vi "Read Boolean Configuration.vi"(8 "error in (no error)":errorcluster, 9 "Default If Not Found":bool, 10 "Name":string, 11 "database-configuration in":refnum<class "configuration-database.lvclass">) -> (0 "error out":errorcluster, 1 "Not Found?":bool, 2 "Value":bool, 3 "database-configuration out":refnum<class "configuration-database.lvclass">)   [LabVIEW 2020, in "configuration-database.lvlib" / "configuration-database.lvclass"]
uses:
  configuration-database.lvclass
  configuration-database.lvclass/configuration-database.ctl
  bde3cf0d-0dad-4714-9e3b-43a1a7f5128d.vi
  bde3cf0d-0dad-4714-9e3b-43a1a7f5128d.vi/28ee1364-3f60-465d-b3c8-c72d5691017c.vi
  <vilib>/Utility/error.llb/Error Cluster From Error Code.vi
  IConfigDBQueries/IConfigurationDatabaseQueries.lvclass
  externals/database-interface/IDatabase/IDatabase/IDatabase.lvclass
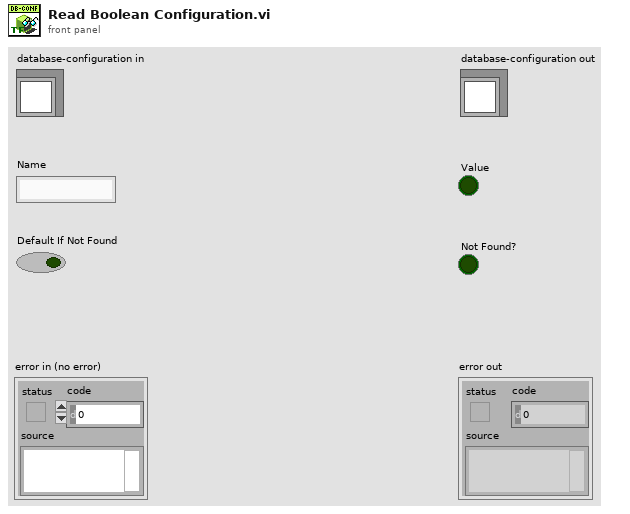
[diagram p1: front panel]
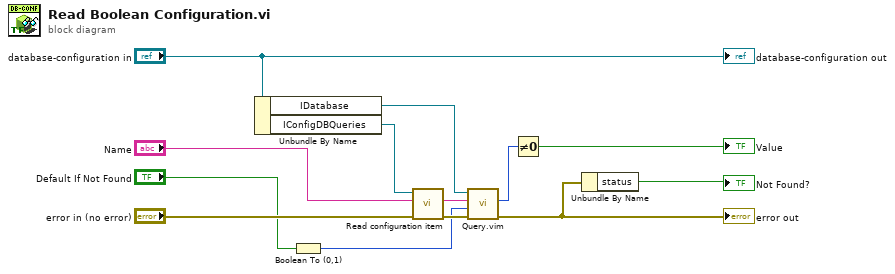
[diagram p0: block diagram]
diagram:
  n1 = Unbundle By Name("database-configuration in") -> ("IDatabase"=w12:refnum<class "IDatabase.lvclass">, "IConfigDBQueries"=w13:refnum<class "IConfigurationDatabaseQueries.lvclass">)
  n2 = Boolean To (0,1)(Boolean="Default If Not Found") -> (0, 1=w5:i16)
  n3 = call-dynamic "Read configuration item.vi"("error in (no error)"="error in (no error)", "configuration item"="Name", "IConfigDBQueries in"=w13) -> ("error out"=w11:errorcluster, "result"=w10:string)  [unwired: 7 in]
  n4 = call "Query.vim"("error in (no error)"=w11, "Type and Default"=w5, "Query string"=w10, "IDatabase in"=w12) -> ("error out"=w2:errorcluster, "Result"=w4:i32)  [unwired: 5 in, 1 out]
  "error out" <- w2
  n5 = Not Equal To 0?(x=w4) -> (x != 0?=→"Value":bool)
  n6 = Unbundle By Name(w2) -> ("status"=→"Not Found?":bool)
  "database-configuration out" <- "database-configuration in"
